vi "Day 5-2.vi"() -> ()   [LabVIEW 2019, in "Day 5.lvlib"]
uses:
  Day 5.lvlib
panel:
  out "dimension size":i32
  out "Array":i32[][](array[numeric])
  out "Yf":i32[](array[numeric])
  out "Xf":i32[](array[numeric])
  out "Yi":i32[](array[numeric])
  out "Xi":i32[](array[numeric])
  in  "String":string
  # "18540"
  # "19995"
  # "19949"
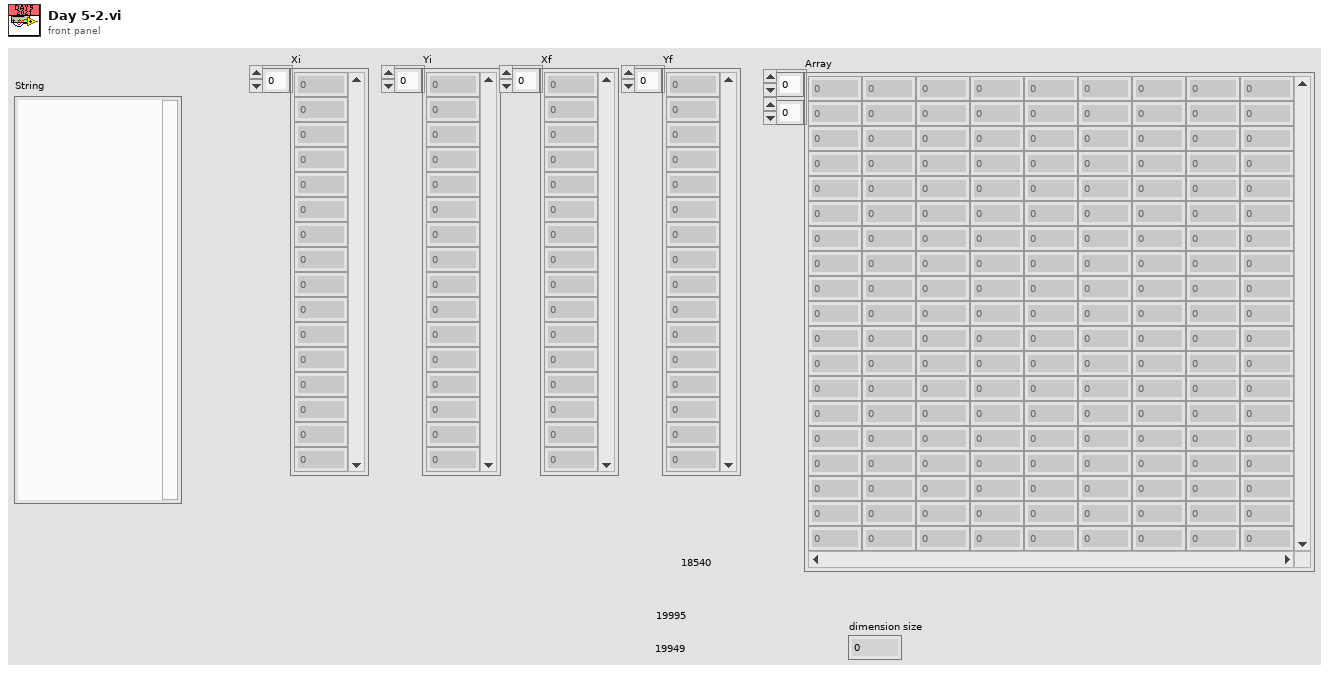
[diagram p1: front panel]
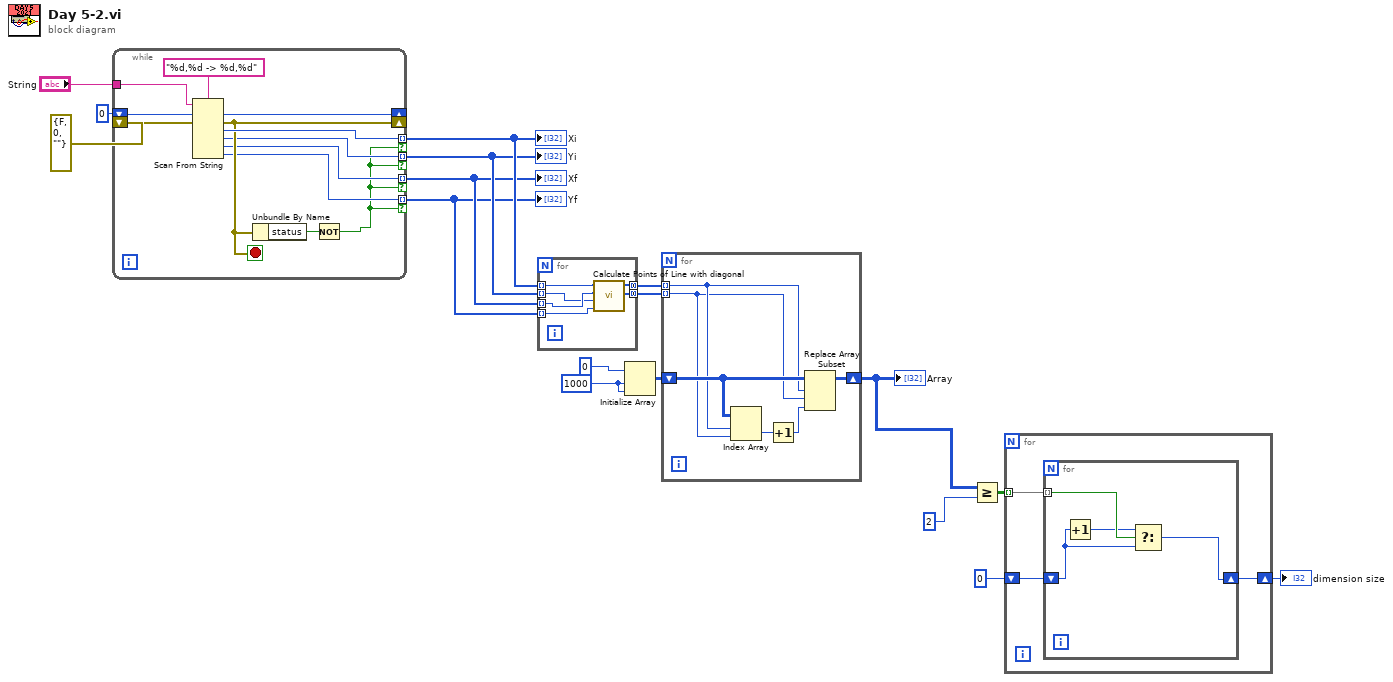
[diagram p0: block diagram]
diagram:
  w13 = 1000 ("dimension size")
  n1 = while {
    tunnel: [w27] -> w12 mode=indexing if=w18
    tunnel: "String" -> [w29]
    shift-right: [w24] -> _
    shift-left: u32 0 -> [w26]
    shift-right: [w23] -> _
    shift-left: errorcluster {"status"=FALSE, "code"=0, "source"=""} ("error IO") -> [w25]
    tunnel: [w21] -> w11 mode=indexing if=w18
    tunnel: [w20] -> w10 mode=indexing if=w18
    tunnel: [w19] -> w9 mode=indexing if=w18
    stop <- w23 stop-if-true
    n2 = Scan From String(format string="%d,%d -> %d,%d", input string=w29, initial scan location=w26, error in=w25) -> (offset past scan=w24:u32, error out=w23:errorcluster, output 1=w27:i32, output 2=w21:i32, output 3=w20:i32, output 4=w19:i32)  [unwired: 4 in, 1 out]
    n3 = Unbundle By Name(w23) -> ("status"=w22:bool)
    n4 = Not(x=w22) -> (.not. x?=w18:bool)
  }
  "Xi" <- w12
  "Yi" <- w11
  "Xf" <- w10
  "Yf" <- w9
  n5 = for {
    tunnel: w12 -> [w35] mode=indexing
    tunnel: w11 -> [w32] mode=indexing
    tunnel: w10 -> [w34] mode=indexing
    tunnel: w9 -> [w33] mode=indexing
    tunnel: [w31] -> w8 mode=concatenating
    tunnel: [w30] -> w7 mode=concatenating
    n6 = call "Calculate Points of Line with diagonal.vi"("Yf"=w33, "Yi"=w32, "Xf"=w34, "Xi"=w35) -> ("Y Points"=w30:i32[], "X Points"=w31:i32[])  [unwired: 6 in]
  }
  n7 = Initialize Array(0 ("dimension size"), w13, w13) -> (w6:i32[][])
  n8 = for {
    tunnel: w8 -> [w40] mode=indexing
    tunnel: w7 -> [w39] mode=indexing
    shift-right: [w36] -> w1
    shift-left: w6 -> [w41]
    n9 = Index Array(array=w41, index (row)=w40, index (col)=w39) -> (element=w38:i32)
    n10 = Increment(x=w38) -> (x+1=w37:i32)
    n11 = Replace Array Subset(array=w41, new element=w37, index (row)=w40, index (col)=w39) -> (w36:i32[][])
  }
  "Array" <- w1
  n12 = Greater Or Equal?(x=w1, y=2 ("dimension size")) -> (x >= y?=w4:bool[][])
  n13 = for {
    tunnel: w4 -> [w44] mode=indexing
    shift-right: [w42] -> w2
    shift-left: 0 ("dimension size") -> [w43]
    n14 = for {
      tunnel: w44 -> [w48] mode=indexing
      shift-right: [w47] -> w42
      shift-left: w43 -> [w45]
      n15 = Increment(x=w45) -> (x+1=w46:i32)
      n16 = Select(t=w46, s=w48, f=w45) -> (s? t:f=w47:i32)
    }
  }
  "dimension size" <- w2
